vi "pf_Set_Camera_Property_Bool.vi"(8 "error in (no error)":errorcluster, 9 "Property Value":bool, 10 "Property Name":string, 11 "IMAQ Session in":refnum<k11>) -> (0 "error out":errorcluster, 2 "Property Name out":string, 3 "IMAQ Session out":refnum<k11>)   [LabVIEW 2025, in "Photonfocus_Toolkit.lvlib"]
doc: "Sets the value of a Boolean type property."
uses:
  Photonfocus_Toolkit.lvlib
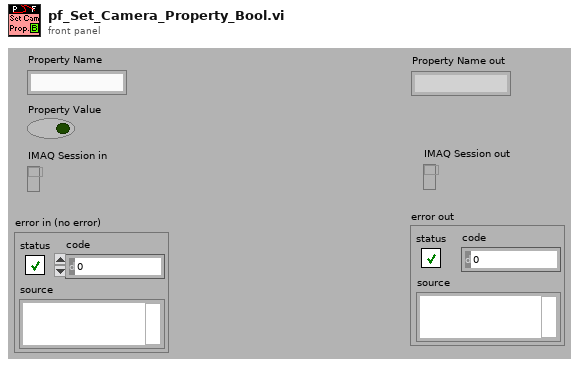
[diagram p1: front panel]
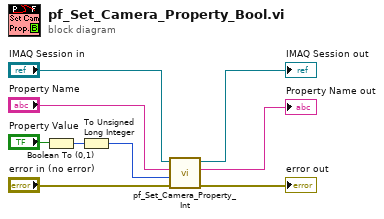
[diagram p0: block diagram]
diagram:
  n1 = Boolean To (0,1)(Boolean="Property Value") -> (0, 1=w3:i16)
  n2 = To Unsigned Long Integer(number=w3) -> (unsigned 32bit integer=w2:u32)
  n3 = call "pf_Set_Camera_Property_Int.vi"("error in (no error)"="error in (no error)", "Property Value"=w2, "Property Name"="Property Name", "IMAQ Session in"="IMAQ Session in") -> ("error out"=→"error out":errorcluster, "Property Name out"=→"Property Name out":string, "IMAQ Session out"=→"IMAQ Session out":refnum<k11>)  [unwired: 5 out]
